vi "Set Help.vi"(8 "error in (no error)":errorcluster, 10 "Help":refnum<class "Data.lvclass">, 11 "Data in":refnum<class "Data.lvclass">) -> (0 "error out":errorcluster, 3 "Data out":refnum<class "Data.lvclass">)   [LabVIEW 2015, in "MDSplus.lvlib" / "Data.lvclass"]
doc: "Set the Help field for this Data instance."
uses:
  Data.lvclass
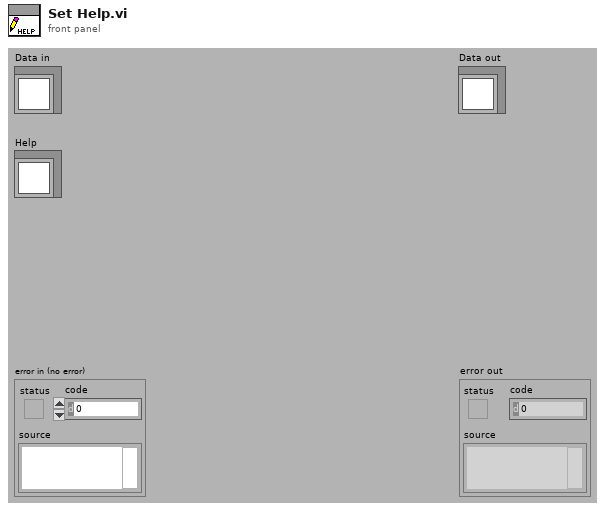
[diagram p1: front panel]
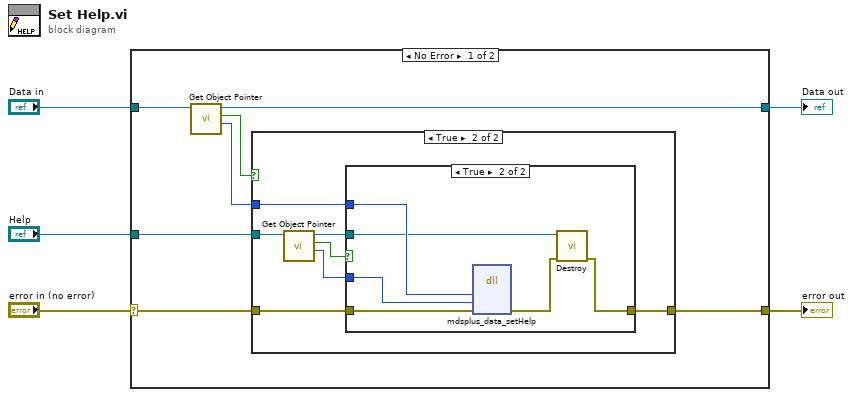
[diagram p0: block diagram]
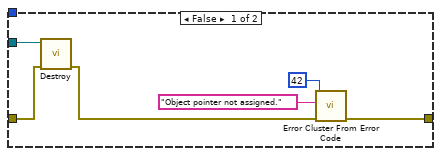
[diagram p2: hidden frame]
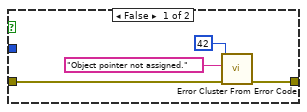
[diagram p3: hidden frame]
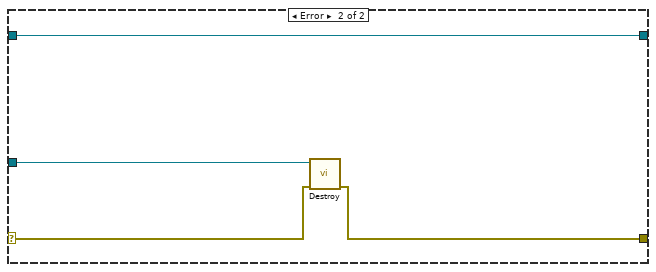
[diagram p4: hidden frame]
diagram:
  n1 = case shown="No Error" "error in (no error)" {
    selector: "error in (no error)" -> [w8 w37]
    tunnel: [w7 w36] -> w4
    tunnel: [w6 w39] -> w2
    tunnel: "Data in" -> [w12 w39]
    tunnel: "Help" -> [w11 w38]
    frame No Error {
      n2 = call-dynamic "Get Object Pointer.vi"("Data in"=w12) -> ("Object Pointer"=w9:i64, "Assigned object pointer?"=w10:bool, "Data out"=w6:refnum<class "Data.lvclass">)  [unwired: 8 in]
      n3 = case shown="True" w10 {
        tunnel: w11 -> [w15 w25]
        tunnel: w9 -> [_ w22]
        tunnel: w8 -> [w14 w21]
        tunnel: [w16 w20] -> w7
        frame False {
          n4 = call-dynamic "Destroy.vi"("error in (no error)"=w14, "Data in"=w15) -> ("error out"=w13:errorcluster)  [unwired: 9 in]
          n5 = call <vilib>:"Error Cluster From Error Code.vi"("error in (no error)"=w13, "error message (\"\")"="Object pointer not assigned." ("error message (\"\")"), "error code (0)"=42) -> ("error out"=w16:errorcluster)  [unwired: 6 in]
        }
        frame True {
          n6 = call-dynamic "Get Object Pointer.vi"("Data in"=w25) -> ("Object Pointer"=w23:i64, "Assigned object pointer?"=w24:bool, "Data out"=w19:refnum<class "Data.lvclass">)  [unwired: 8 in]
          n7 = case shown="True" w24 {
            tunnel: w23 -> [_ w34]
            tunnel: w22 -> [_ w35]
            tunnel: w21 -> [w27 w33]
            tunnel: [w26 w30] -> w20
            tunnel: w19 -> [_ w32]
            frame False {
              n8 = call <vilib>:"Error Cluster From Error Code.vi"("error in (no error)"=w27, "error message (\"\")"="Object pointer not assigned." ("error message (\"\")"), "error code (0)"=42) -> ("error out"=w26:errorcluster)  [unwired: 6 in]
            }
            frame True {
              n9 = dll-call lib="MDSobjectsLVShr" fn="mdsplus_data_setHelp"("lvDataPtr"=w35, "lvDataPtrIn"=w34, "error"=w33) -> ("error"=w31:errorcluster)  [unwired: 6 in, 2 out]
              n10 = call-dynamic "Destroy.vi"("error in (no error)"=w31, "Data in"=w32) -> ("error out"=w30:errorcluster)  [unwired: 9 in]
            }
          }
        }
      }
    }
    frame Error {
      n11 = call-dynamic "Destroy.vi"("error in (no error)"=w37, "Data in"=w38) -> ("error out"=w36:errorcluster)  [unwired: 9 in]
    }
  }
  "error out" <- w4
  "Data out" <- w2
